vi "walk out.vi"(0 "Number of sets of steps":i32=6, 1 "Walk out number steps":u16=10, 2 "Walk out Amplitude (V)":sgl=320.0) -> ()   [LabVIEW 2021]
uses:
  <userlib>/Nanonis Prog Interface V5/Nanonis Prog Interface.lvlib
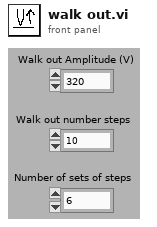
[diagram p1: front panel]
types:
  T1 = enum8{"Group 1", "Group 2", "Group 3", "Group 4", "Group 5", "Group 6"}
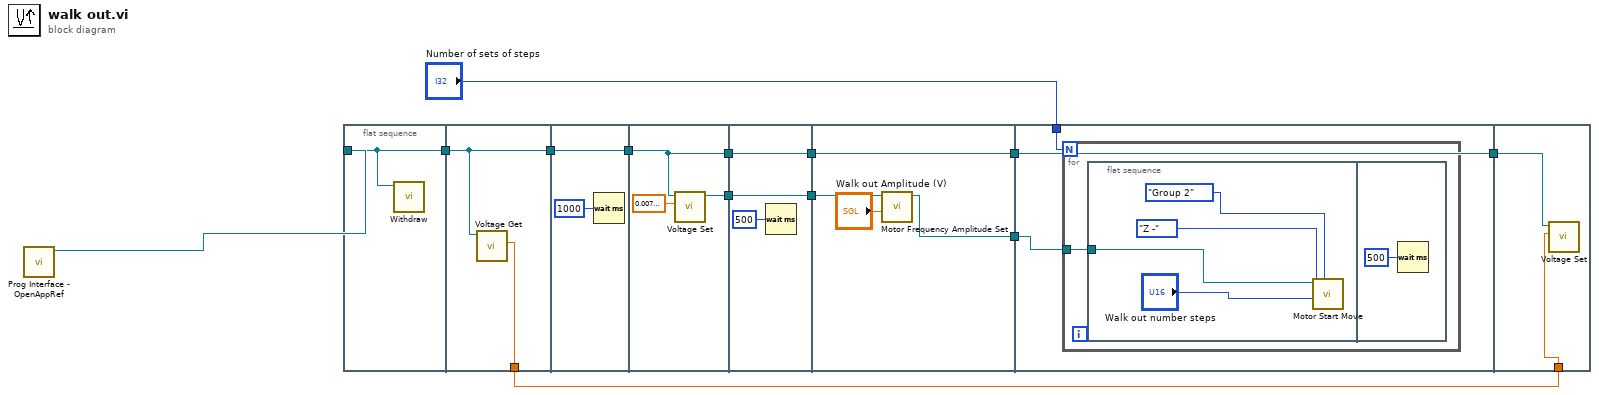
[diagram p0: block diagram]
diagram:
  n1 = call <userlib>:"Prog Interface - OpenAppRef.vi"() -> ("Application reference"=w13:refnum<vi>)  [unwired: 6 in, 1 out]
  n2 = flat-sequence {
    tunnel: [w14] -> w12
    tunnel: w13 -> [w14]
    tunnel: w12 -> [w16]
    tunnel: [w16] -> w11
    tunnel: [w15] -> w1
    tunnel: w11 -> [w18]
    tunnel: [w18] -> w10
    tunnel: [w20] -> w9
    tunnel: w10 -> [w19]
    tunnel: [w19] -> w8
    tunnel: w9 -> [w24]
    tunnel: [w24] -> w7
    tunnel: [w22] -> w6
    tunnel: w8 -> [w22]
    tunnel: w7 -> [w28]
    tunnel: [w27] -> w5
    tunnel: [w25] -> w4
    tunnel: w6 -> [w25]
    tunnel: w5 -> [w31]
    tunnel: "Number of sets of steps" -> [w30]
    tunnel: [w29] -> w3
    tunnel: w4 -> [w29]
    tunnel: w3 -> [w39]
    tunnel: w1 -> [w38]
    frame #0 {
      n3 = call <userlib>:"Withdraw.vi"("Application ref in"=w14) -> ()  [unwired: 9 in, 2 out]
    }
    frame #1 {
      n4 = call <userlib>:"Voltage Get.vi"("Application ref in"=w16) -> ("Bias (V)"=w15:sgl)  [unwired: 8 in, 2 out]
    }
    frame #2 {
      n5 = Wait (ms)(milliseconds to wait=u32 1000) -> ()  [unwired: 1 out]
    }
    frame #3 {
      n6 = call <userlib>:"Voltage Set.vi"("Bias (V)"=sgl 0.007, "Application ref in"=w19) -> ("Application ref out"=w20:refnum<vi>)  [unwired: 8 in, 1 out]
    }
    frame #4 {
      n7 = Wait (ms)(milliseconds to wait=u32 500) -> ()  [unwired: 1 out]
    }
    frame #5 {
      n8 = call <userlib>:"Motor Frequency Amplitude Set.vi"("Amplitude (V) (NaN=no change)"="Walk out Amplitude (V)", "Application ref in"=w28) -> ("Application ref out"=w27:refnum<vi>)  [unwired: 8 in, 1 out]
    }
    frame #6 {
      n9 = for {
        N: w30 -> [_]
        tunnel: w31 -> [w32]
        n10 = flat-sequence {
          tunnel: w32 -> [w34]
          frame #0 {
            n11 = call <userlib>:"Motor Start Move.vi"("Group"=T1."Group 2", "Number of steps"="Walk out number steps", "Direction"=enum16{"X +", "X -", "Y +", "Y -", "Z +", "Z -"}."Z -", "Application ref in"=w34) -> ()  [unwired: 5 in, 2 out]
          }
          frame #1 {
            n12 = Wait (ms)(milliseconds to wait=u32 500) -> ()  [unwired: 1 out]
          }
        }
      }
    }
    frame #7 {
      n13 = call <userlib>:"Voltage Set.vi"("Bias (V)"=w38, "Application ref in"=w39) -> ()  [unwired: 8 in, 2 out]
    }
  }
